vi "Kafka_CloseProducer.vi"(8 "error in (no error)":errorcluster, 11 "Producer Handle":string="localhost:9092") -> (0 "error out":errorcluster, 3 "Producer Handle":string)   [LabVIEW 2019]
uses:
  VS2017/KafkaLVLib/x64/Debug/KafkaLVLib.dll
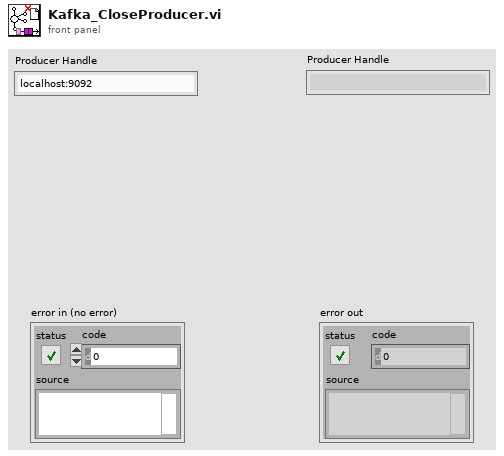
[diagram p1: front panel]
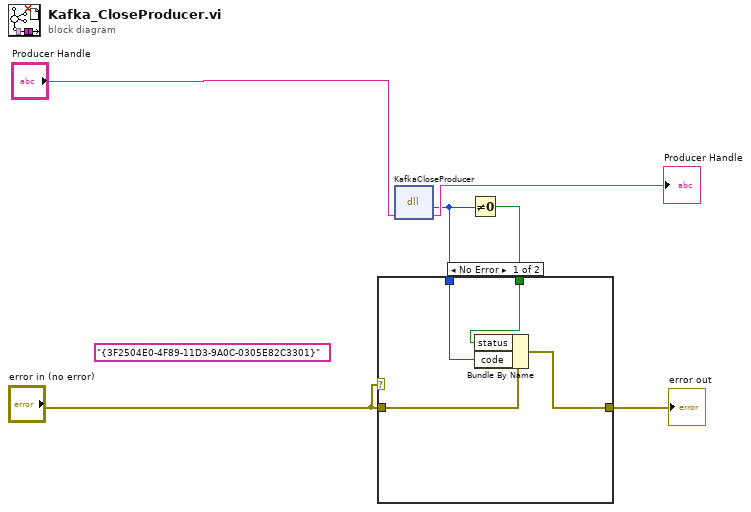
[diagram p0: block diagram]
diagram:
  (unwired) "{3F2504E0-4F89-11D3-9A0C-0305E82C3301}" ("consumerHandle")
  n1 = dll-call lib="C:/Users/schandho/OneDrive - National Instruments/Research/Virtualization/SemiADV/KafkaLVLib/VS2017/KafkaLVLib/x64/Debug/KafkaLVLib.dll" fn="KafkaCloseProducer"("consumerhandle"="Producer Handle") -> ("error"=w2:i32, "consumerhandle"=→"Producer Handle":string)  [unwired: 3 in, 2 out]
  n2 = Not Equal To 0?(x=w2) -> (x != 0?=w3:bool)
  n3 = case shown="No Error" "error in (no error)" {
    tunnel: "error in (no error)" -> [w10 w11]
    tunnel: [w9 w11] -> w5
    tunnel: w3 -> [w8 _]
    tunnel: w2 -> [w7 _]
    frame No Error {
      n4 = Bundle By Name(cluster=w10, "status"=w8, "code"=w7) -> (w9:errorcluster)
    }
    frame Error {
    }
  }
  "error out" <- w5
